vi "Motor temperature.vi"() -> ()   [LabVIEW 2016]
uses:
  <vilib>/CANopenLib/CANOPEN.llb/CANopen SDO Create.vi
  Get Motor Temperature.vi
panel:
  in  "Node ID":u8=2
  out "SDO object out":refnum<k20>
  out "U8 data":u8
  out "completion code":u32 format="%.0x"
  out "error out":errorcluster
  in  "timeout (1s)":dbl=1.0 min=0.0
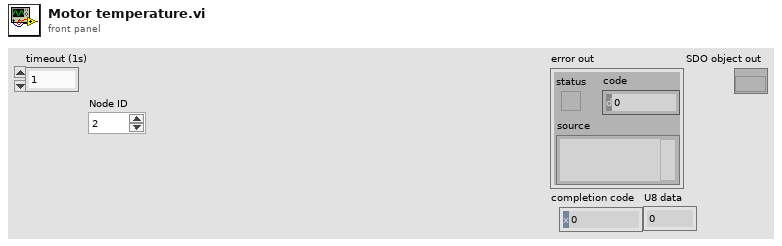
[diagram p1: front panel]
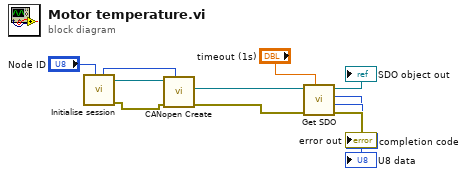
[diagram p0: block diagram]
diagram:
  n1 = call "Initialise session.vi"("Node ID"="Node ID") -> ("error out"=w10:errorcluster, "interface object out"=w11:refnum<k20>, "Used Node ID"=w1:u8)  [unwired: 8 in]
  n2 = call-poly <vilib>:"CANopen Create.vi"("node-ID"=w1, "error in (no error)"=w10, "interface object in"=w11) -> ("error out"=w8:errorcluster, "SDO object out"=w9:refnum<k20>)  [unwired: 6 in, 1 out]
  n3 = call-poly "Get SDO.vi"("timeout (1s)"="timeout (1s)", "error in (no error)"=w8, "SDO object in"=w9) -> ("error out"=→"error out":errorcluster, "completion code"=→"completion code":u32, "U8 data"=→"U8 data":u8, "SDO object out"=→"SDO object out":refnum<k20>)  [unwired: 5 in]
